vi "Get Target Position.vi"(8 "error in":errorcluster) -> (0 "error out":errorcluster, 2 "target y (mm)":dbl, 3 "target x (mm)":dbl)   [LabVIEW 2017, in "Game.lvlib"]
uses:
  Game.lvlib
  Public TypeDefs/Target Position.ctl
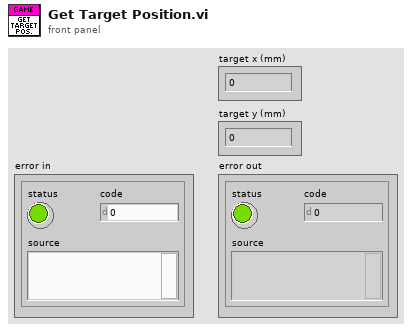
[diagram p1: front panel]
types:
  T1 = typedef "Game.lvlib/Target Position.ctl" = cluster{"x (mm)":dbl, "y (mm)":dbl}
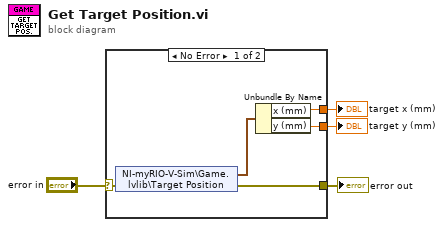
[diagram p0: block diagram]
diagram:
  n1 = case shown="No Error" "error in" {
    selector: "error in" -> [w9 w10]
    tunnel: [w8 w10] -> w3
    tunnel: [w6 _] -> w2
    tunnel: [w5 _] -> w1
    frame No Error {
      n2 = shared-variable "NI-myRIO-V-Sim\\Game.lvlib\\Target Position"(error in=w9) -> (w7:T1, error out=w8:errorcluster)
      n3 = Unbundle By Name(w7) -> ("x (mm)"=w6:dbl, "y (mm)"=w5:dbl)
    }
    frame Error {
    }
  }
  "error out" <- w3
  "target x (mm)" <- w2
  "target y (mm)" <- w1
